vi "setLabelProperties.vi"(6 "visible":bool, 8 "error in (no error)":errorcluster, 10 "label":string, 11 "Wire in":refnum<class "Wire.lvclass">) -> (0 "error out":errorcluster, 3 "Wire in":refnum<class "Wire.lvclass">)   [LabVIEW 2023, in "TLC_Scripto.lvlib" / "Wire.lvclass"]
uses:
  Wire.lvclass
  Wire.lvclass/Wire.ctl
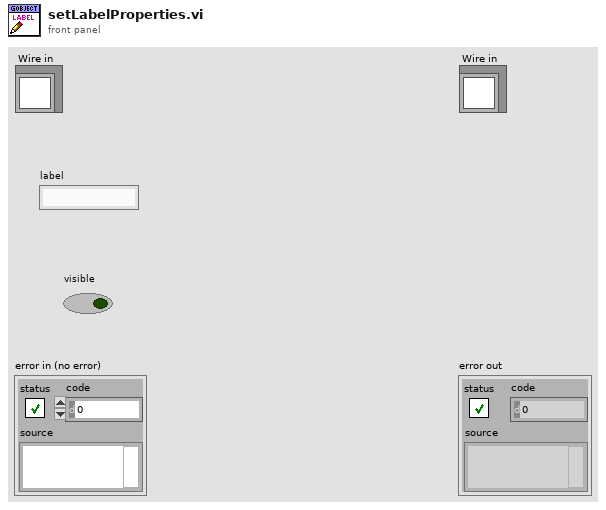
[diagram p1: front panel]
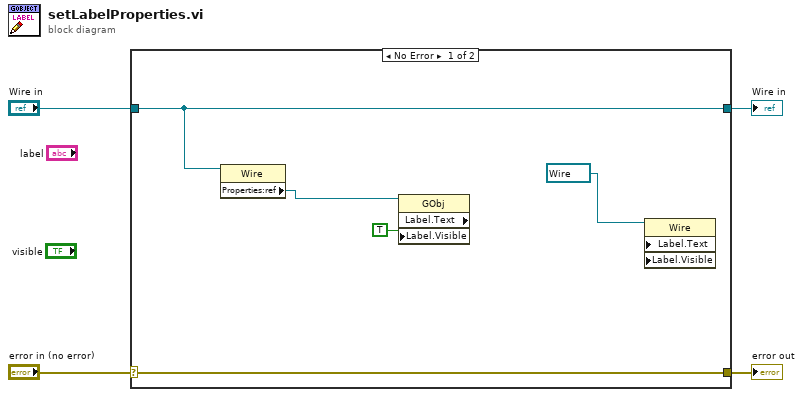
[diagram p0: block diagram]
diagram:
  n1 = case shown="No Error" "error in (no error)" {
    selector: "error in (no error)" -> [w10 w12]
    tunnel: [w10 w12] -> w3
    tunnel: [w7 w11] -> w1
    tunnel: "Wire in" -> [w7 w11]
    frame No Error {
      n2 = property class="Wire"(reference=w7) -> ("Properties:ref"=w6:refnum<vi>)  [unwired: 1 in, 2 out]
      n3 = property class="GObj"(reference=w6, "Label.Visible"=TRUE) -> ("Label.Text"=w9)  [unwired: 1 in, 2 out]
      n4 = property class="Wire" props=["Label", "Text", "Label", "Visible"](reference=refnum<vi> refnum ("ref")) -> ()  [unwired: 3 in, 2 out]
    }
    frame Error {
    }
  }
  "error out" <- w3
  "Wire in" <- w1
